vi "1762PointUpProgram.vi"() -> ()   [LabVIEW 2012]
uses:
  <vilib>/Utility/file.llb/Write To Spreadsheet File (DBL).vi
panel:
  out "digital waveform out 3":digitalwaveform(waveform)={"t0"=timestamp(0 s since 1904-01-01), "dt"=1e-07, "Y"={"transitions"=[0, 20000, 21001, 21501, 22501, 42500], "data"=[[1, 1, 0, 0], [0, 0, 0, 0], [0, 0, 0, 1], [0, 0, 0, 0], [1, 1, 0, 0], [1, 1, 0, 0]]}, "error"={"status"=FALSE, "code"=37421928, "source"=""}}
  out "10xwindow":i32
  out "10xdiscr":dbl
  out "DARK?":i32(graph)
  out "Counts":i32
  out "DARK?":bool
  out "PMT Counts":i32(graph)
  in  "PMT sample time":dbl=0.05
  out "Counts after 1762":i32=57
  out "OuterLoop":i32=101
  out "InnerLoop":i32=19
  out "Frequency Step Size":dbl=10000.0
  out "Bright Events":dbl
  in  "Discriminator Level\n (Bright/Dark)":i32=28
  out "digital waveform out 2":digitalwaveform(waveform)={"t0"=timestamp(0 s since 1904-01-01), "dt"=1e-07, "Y"={"transitions"=[0, 20000, 21001, 21501, 22501, 42500], "data"=[[1, 1, 0, 0], [0, 0, 0, 0], [0, 0, 0, 1], [0, 0, 0, 0], [1, 1, 0, 0], [1, 1, 0, 0]]}, "error"={"status"=FALSE, "code"=37421928, "source"=""}}
  in  "1762 pulse length (units of 1 us)":dbl=50.0
  in  "Comment":string="SPAOM, DPAOM = 77 MHz"
  in  "B Field":dbl=2.26
  in  "Power":dbl
  in  "Rerun BG Every\nnth freq point":dbl=20.0
  in  "PMT sample time":dbl=0.05
  out "Counts finding bright ion":dbl=39.0
  in  "BG Cutoff Limit":dbl=38.0
  in  "Runs per data point":dbl=50.0
  in  "Low Freq":dbl(slide)=83600000.0 min=50000000.0 max=120000000.0 step=1000.0 scale=80000000.0..90000000.0 scale format="%#.5f"
  in  "High Freq":dbl(slide)=84100000.0 min=50000000.0 max=120000000.0 step=1000.0 scale=80000000.0..90000000.0 scale format="%#.0f"
  out "Cur Freq":dbl=85984000.0 format="%#_8f"
  out "Path":path=path "c:/data/1762 Scans/2014-05-20_19-16-05_1762scanWithPumping.txt"
  out "Frequency Scan":cluster{dbl, dbl}[](graph)=[{87004000.0, 1.0}, {86994000.0, 1.0}, {86984000.0, 1.0}, {86974000.0, 1.0}, {86964000.0, 1.0}, {86954000.0, 1.0}, {86944000.0, 1.0}, {86934000.0, 1.0}, {86924000.0, 1.0}, {86914000.0, 1.0}, {86904000.0, 1.0}, {86894000.0, 1.0}, {86884000.0, 1.0}, {86874000.0, 1.0}, {86864000.0, 1.0}, {86854000.0, 1.0}, {86844000.0, 1.0}, {86834000.0, 1.0}, {86824000.0, 1.0}, {86814000.0, 1.0}, {86804000.0, 1.0}, {86794000.0, 1.0}, {86784000.0, 1.0}, {86774000.0, 1.0}, {86764000.0, 1.0}, {86754000.0, 1.0}, {86744000.0, 1.0}, {86734000.0, 1.0}, {86724000.0, 1.0}, {86714000.0, 1.0}, {86704000.0, 1.0}, {86694000.0, 1.0}, {86684000.0, 1.0}, {86674000.0, 1.0}, {86664000.0, 1.0}, {86654000.0, 1.0}, {86644000.0, 1.0}, {86634000.0, 1.0}, {86624000.0, 1.0}, {86614000.0, 1.0}, {86604000.0, 1.0}, {86594000.0, 1.0}, {86584000.0, 1.0}, {86574000.0, 1.0}, {86564000.0, 1.0}, {86554000.0, 1.0}, {86544000.0, 1.0}, {86534000.0, 1.0}, {86524000.0, 1.0}, {86514000.0, 1.0}, {86504000.0, 1.0}, {86494000.0, 1.0}, {86484000.0, 1.0}, {86474000.0, 1.0}, {86464000.0, 1.0}, {86454000.0, 1.0}, {86444000.0, 1.0}, {86434000.0, 1.0}, {86424000.0, 1.0}, {86414000.0, 1.0}, {86404000.0, 1.0}, {86394000.0, 1.0}, {86384000.0, 1.0}, {86374000.0, 1.0}, {86364000.0, 1.0}, {86354000.0, 1.0}, {86344000.0, 1.0}, {86334000.0, 1.0}, {86324000.0, 1.0}, {86314000.0, 1.0}, {86304000.0, 1.0}, {86294000.0, 1.0}, {86284000.0, 1.0}, {86274000.0, 1.0}, {86264000.0, 1.0}, {86254000.0, 1.0}, {86244000.0, 1.0}, {86234000.0, 1.0}, {86224000.0, 1.0}, {86214000.0, 1.0}, {86204000.0, 1.0}, {86194000.0, 1.0}, {86184000.0, 1.0}, {86174000.0, 1.0}, {86164000.0, 1.0}, {86154000.0, 1.0}, {86144000.0, 1.0}, {86134000.0, 1.0}, {86124000.0, 1.0}, {86114000.0, 1.0}, {86104000.0, 1.0}, {86094000.0, 1.0}, {86084000.0, 1.0}, {86074000.0, 1.0}, {86064000.0, 1.0}, {86054000.0, 1.0}, {86044000.0, 1.0}, {86034000.0, 1.0}, {86024000.0, 1.0}, {86014000.0, 1.0}, {86004000.0, 1.0}, {85994000.0, 1.0}]
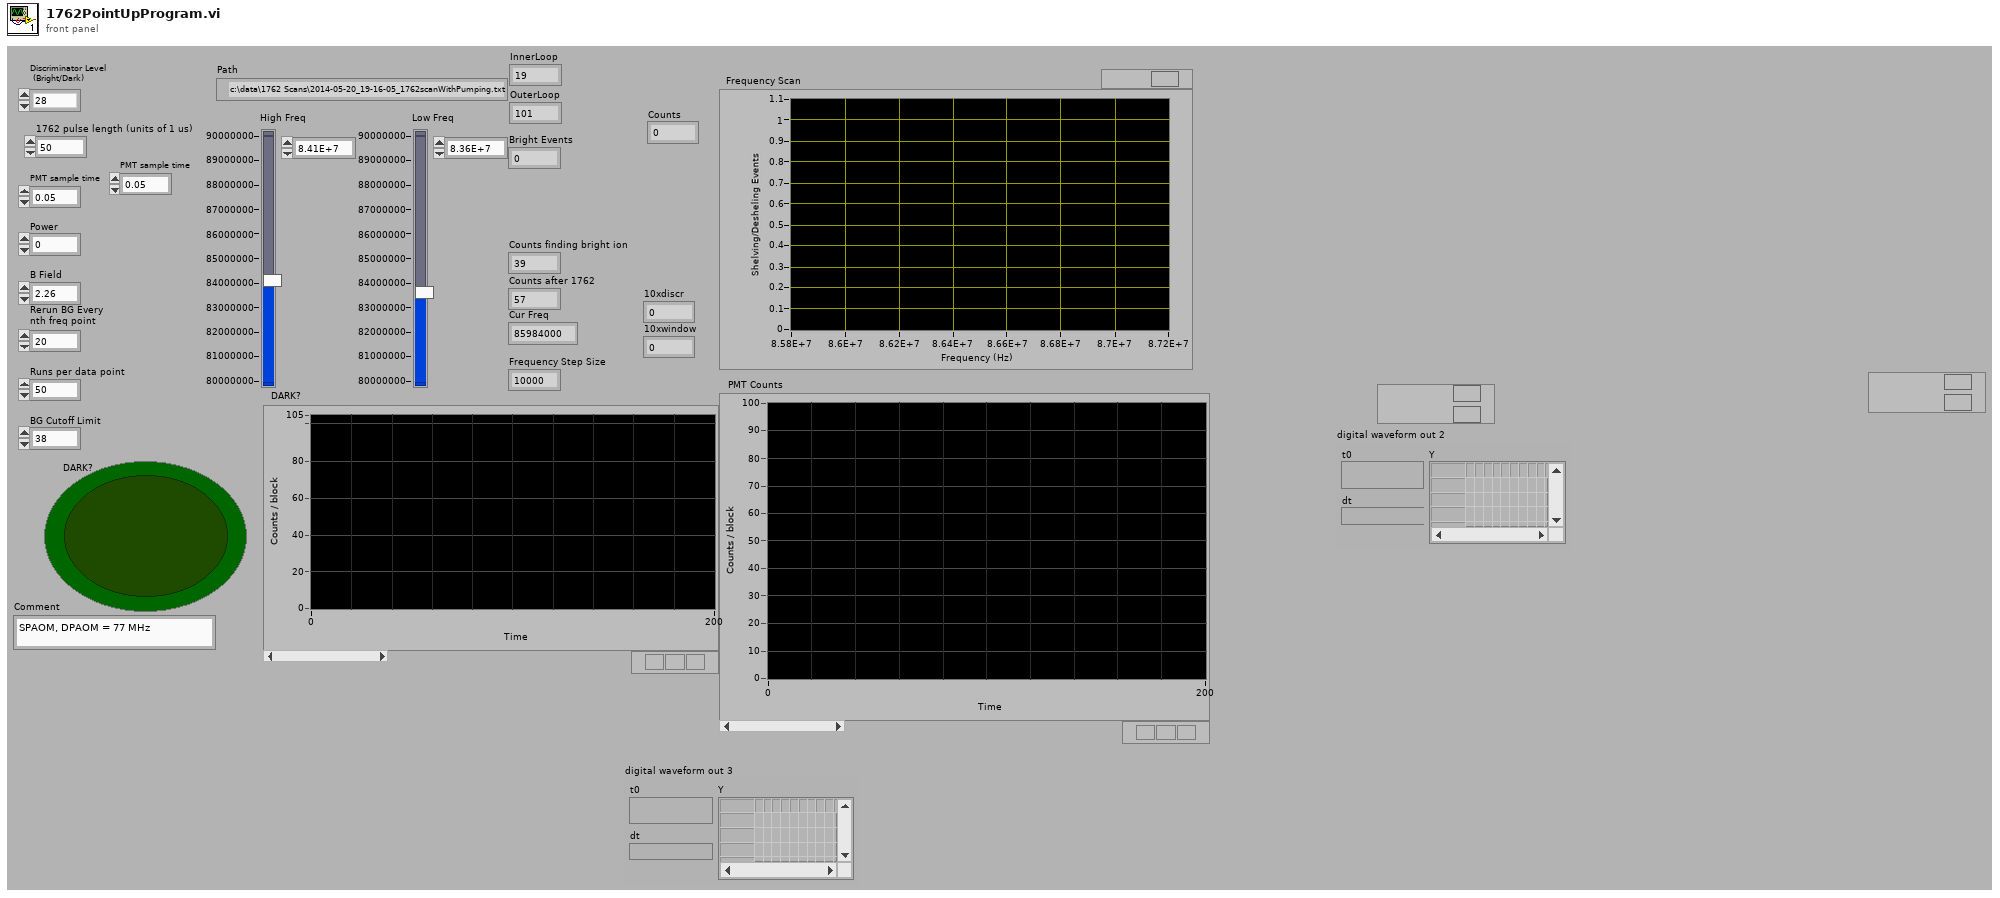
[diagram p1: front panel]
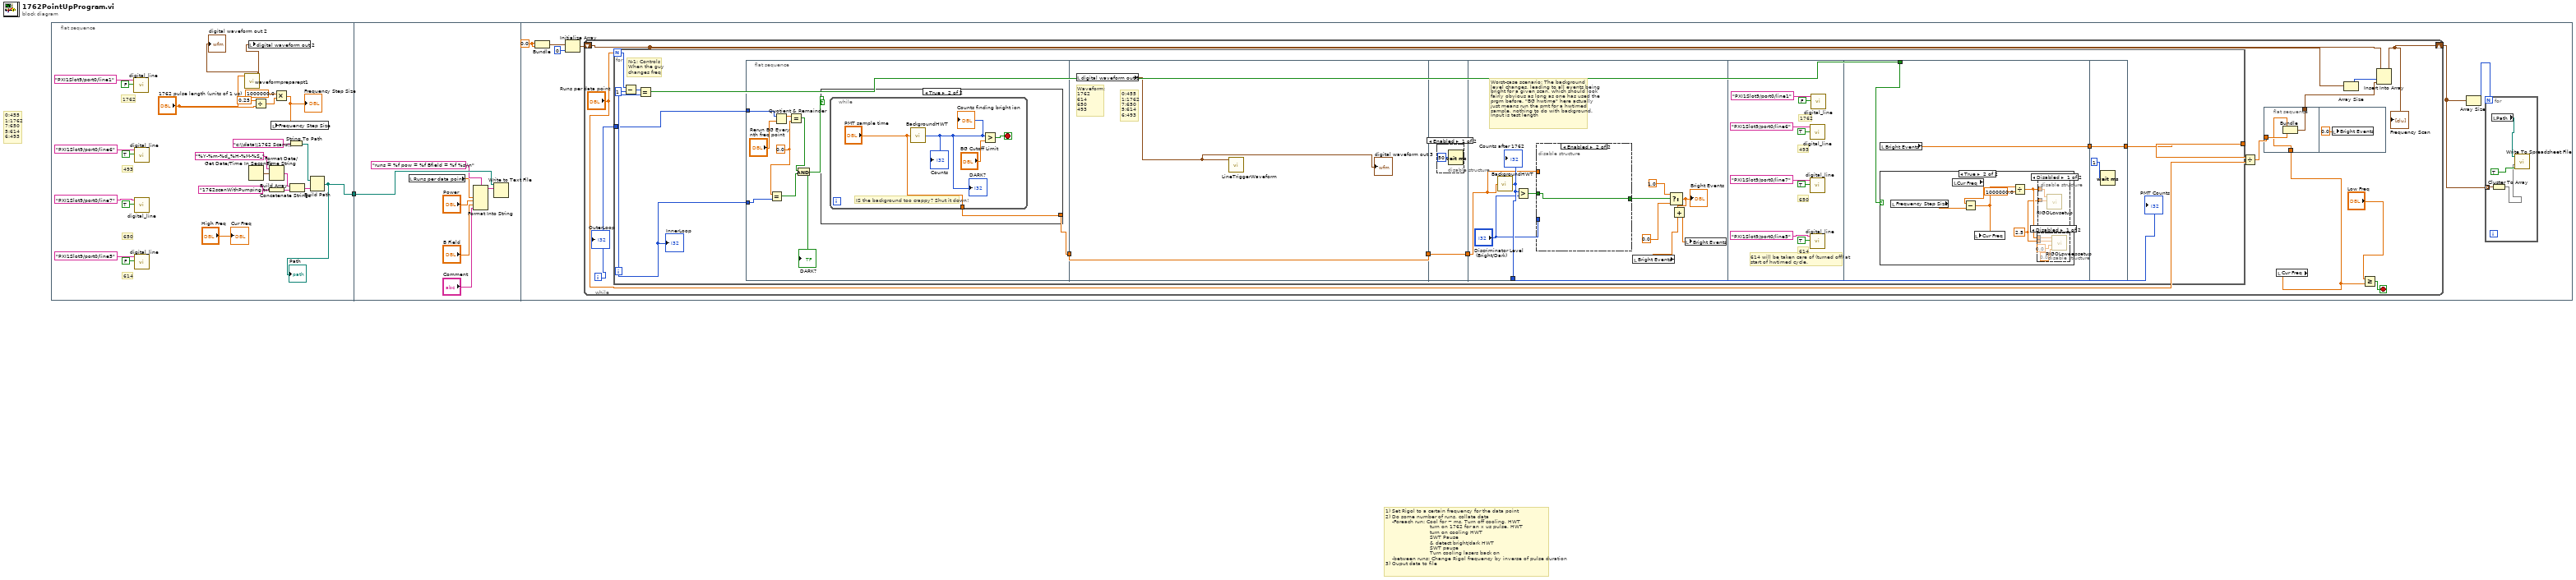
[diagram p0: block diagram]
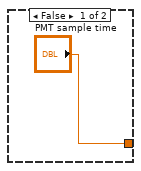
[diagram p2: hidden frame]
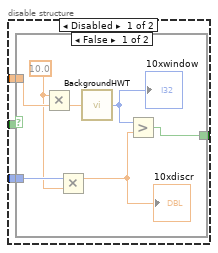
[diagram p4: hidden frame]
diagram:
  # "0:455\n1:1762\n7:650\n5:614\n6:493"
  # "1) Set Rigol to a certain frequency for the data point\n2) Do some number of runs, collate data\n    -Foreach run: Cool for ~ ms, Turn off cooling, HWT\n                           turn on 1762 for an x us pulse, HWT\n                           turn on cooling HWT\n                           SWT Pause\n                           & detect bright/dark HWT\n                           SWT pause\n                           Turn cooling lasers back on \n    -between runs: Change Rigol frequency by inverse of pulse duration\n3) Ouput data to file"
  n1 = flat-sequence {
    tunnel: [w17] -> w1
    tunnel: w1 -> [w32]
    frame #0 {
      # "614"
      # "650"
      # "493"
      # "1762"
      n2 = call "digital_line.vi"("Boolean"=FALSE, "lines"=tag "PXI1Slot9/port0/line1") -> ()  [unwired: 5 in, 1 out]
      n3 = call "digital_line.vi"("Boolean"=TRUE, "lines"=tag "PXI1Slot9/port0/line6") -> ()  [unwired: 5 in, 1 out]
      n4 = call "digital_line.vi"("Boolean"=TRUE, "lines"=tag "PXI1Slot9/port0/line7") -> ()  [unwired: 5 in, 1 out]
      n5 = call "digital_line.vi"("Boolean"=FALSE, "lines"=tag "PXI1Slot9/port0/line5") -> ()  [unwired: 5 in, 1 out]
      n6 = call "waveformpreparept1.vi"("1762 pulse length (units of 1 us)"="1762 pulse length (units of 1 us)") -> ("digital waveform out 2"=w2:digitalwaveform)  [unwired: 8 in]
      "digital waveform out 2" <- w2
      n7 = local write "digital waveform out 2"(w2) -> ()
      n8 = Get Date/Time In Seconds() -> (seconds since 1Jan1904=w19:timestamp)
      n9 = Divide(x=0.25, y="1762 pulse length (units of 1 us)") -> (x/y=w5:dbl)
      n10 = Format Date/Time String(time format string (%c)="%Y-%m-%d_%H-%M-%S_", seconds (now)=w19) -> (date/time string=w21:string)  [unwired: 1 in]
      n11 = Build Array("1762scanWithPumping.txt") -> (w24:string[])
      n12 = Multiply(x=1000000.0, y=w5) -> (x*y=w6:dbl)
      "Frequency Step Size" <- w6
      n13 = local write "Frequency Step Size"(w6) -> ()
      n14 = String To Path(string="c:\\data\\1762 Scans\\") -> (path=w25:path)
      n15 = Concatenate Strings(w21, w24) -> (w23:string)
      n16 = Build Path(base path=w25, name or relative path=w23) -> (appended path=w17:path)
      "Path" <- w17
      "Cur Freq" <- "High Freq"
    }
    frame #1 {
      n17 = local read "Runs per data point"() -> (w29:dbl)
      n18 = Format Into String(format string="runs = %f pow = %f Bfield = %f %s\\n", w29, "Power", "B Field", "Comment") -> (resulting string=w30:string)  [unwired: 2 in, 1 out]
      n19 = Write to Text File(file (use dialog)=w32, text=w30) -> ()  [unwired: 2 in, 3 out]
    }
    frame #2 {
      w37 = 0.0
      n20 = Bundle(w37, w37) -> (w38:cluster{dbl, dbl})  [unwired: 1 in]
      n21 = Initialize Array(w38, 0) -> (w35:cluster{dbl, dbl}[])
      n22 = while {
        shift-right: [w49] -> w33
        shift-left: w35 -> [w50]
        i -> [w48]
        stop <- w52 stop-if-true
        n23 = for {
          N: "Runs per data point" -> [w66]
          tunnel: [w65] -> w45
          tunnel: w48 -> [w62]
          i -> [w63]
          # "N-1: Controls\nWhen the guy\nchanges freq"
          n24 = Subtract(x=w66, y=1) -> (x-y=w69:i32)
          n25 = Equal?(x=w69, y=w63) -> (x = y?=w67:bool)
          n26 = flat-sequence {
            tunnel: w63 -> [w76]
            tunnel: w62 -> [w71]
            tunnel: [w70] -> w61
            tunnel: [w86] -> w58
            tunnel: w61 -> [w86]
            tunnel: [w87] -> w59
            tunnel: w58 -> [w87]
            tunnel: w59 -> [w91]
            tunnel: [w93] -> w60
            tunnel: w67 -> [w120]
            tunnel: [w121] -> w64
            tunnel: [w135] -> w65
            tunnel: w64 -> [w135]
            frame #0 {
              w75 = 0.0 ("x")
              n27 = Equal?(x=w75, y=w76) -> (x = y?=w73:bool)
              n28 = Quotient & Remainder(x=w71, y="Rerun BG Every\nnth freq point") -> (x-y*floor(x/y)=w77:dbl)  [unwired: 1 out]
              n29 = Equal?(x=w77, y=w75) -> (x = y?=w74:bool)
              n30 = And(x=w74, y=w73) -> (x .and. y?=w72:bool)
              "DARK?" <- w72
              n31 = case shown="True" w72 {
                tunnel: ["PMT sample time" w80] -> w70
                frame False {
                }
                frame True {
                  n32 = while {
                    tunnel: ["PMT sample time"] -> w80
                    stop <- w83 stop-if-true
                    # "IS the background too crappy? Shut it down!"
                    n33 = call "BackgroundHWT.vi"("Sample Time(seconds)"="PMT sample time") -> ("Counts"=w81:i32)
                    "Counts finding bright ion" <- w81
                    "Counts" <- w81
                    "DARK?" <- w81
                    n34 = Greater?(x=w81, y="BG Cutoff Limit") -> (0:w83:bool)
                  }
                }
              }
            }
            frame #1 {
              # "0:455\n1:1762\n7:650\n5:614\n6:493"
              # "Waveform:\n1762\n614\n650\n493"
              n35 = local read "digital waveform out 2"() -> (w85:digitalwaveform)
              "digital waveform out 3" <- w85
              n36 = call "LineTriggerWaveform.vi"("digital waveform in"=w85) -> ()  [unwired: 11 in]
            }
            frame #2 {
              n37 = disable-structure shown="Enabled" {
                frame Enabled {
                  n38 = Wait (ms)(milliseconds to wait=u32 50) -> ()  [unwired: 1 out]
                }
                frame Disabled {
                }
              }
            }
            frame #3 {
              # "Worst-case scenario: The background\nlevel changes, leading to all events being\nbright for a given scan, which should look\nfairly obvious as long as one has used the\nprgm before. \"BG hwtime\" here actually\njust means run the pmt for a hwtimed\nsample, nothing to do with background.\nInput is test length"
              n39 = call "BackgroundHWT.vi"("Sample Time(seconds)"=w91) -> ("Counts"=w93:i32)
              "Counts after 1762" <- w93
              n40 = Greater?(x=w93, y="Discriminator Level\n (Bright/Dark)") -> (0:w92:bool)
              n41 = disable-structure shown="Enabled" {
                disable-tunnel: w92 -> [w102 w111]
                disable-tunnel: [w101 w111] -> w89
                disable-tunnel: w91 -> [w100 _]
                disable-tunnel: "Discriminator Level\n (Bright/Dark)" -> [w99 _]
                frame Disabled {
                  n42 = case shown="False" w102 {
                    selector: w102 -> [_ w110]
                    tunnel: [w105 w110] -> w101
                    tunnel: w100 -> [w109 _]
                    tunnel: w99 -> [w106 _]
                    frame False {
                      w103 = 10.0 ("x")
                      n43 = Multiply(x=w103, y=w109) -> (x*y=w108:dbl)
                      n44 = Multiply(x=w106, y=w103) -> (x*y=w104:dbl)
                      "10xdiscr" <- w104
                      n45 = call "BackgroundHWT.vi"("Sample Time(seconds)"=w108) -> ("Counts"=w107:i32)
                      "10xwindow" <- w107
                      n46 = Greater?(x=w107, y=w104) -> (0:w105:bool)
                    }
                    frame True {
                    }
                  }
                }
                frame Enabled {
                }
              }
              n47 = local read "Bright Events"() -> (w94:dbl)
              n48 = Select(t=1.0, s=w89, f=0.0) -> (s? t:f=w96:dbl)
              "Bright Events" <- w96
              n49 = Add(x=w96, y=w94) -> (x+y=w95:dbl)
              n50 = local write "Bright Events"(w95) -> ()
            }
            frame #4 {
              # "614 will be taken care of (turned off) at\nstart of hwtimed cycle."
              # "614"
              # "650"
              # "493"
              # "1762"
              n51 = call "digital_line.vi"("Boolean"=TRUE, "lines"=tag "PXI1Slot9/port0/line6") -> ()  [unwired: 5 in, 1 out]
              n52 = call "digital_line.vi"("Boolean"=TRUE, "lines"=tag "PXI1Slot9/port0/line7") -> ()  [unwired: 5 in, 1 out]
              n53 = call "digital_line.vi"("Boolean"=TRUE, "lines"=tag "PXI1Slot9/port0/line5") -> ()  [unwired: 5 in, 1 out]
              n54 = call "digital_line.vi"("Boolean"=FALSE, "lines"=tag "PXI1Slot9/port0/line1") -> ()  [unwired: 5 in, 1 out]
            }
            frame #5 {
              n55 = case shown="True" w120 {
                frame False {
                }
                frame True {
                  w122 = 2.5 ("Amplitude (Vpp)")
                  n56 = local read "Frequency Step Size"() -> (w126:dbl)
                  n57 = local read "Cur Freq"() -> (w127:dbl)
                  n58 = Subtract(x=w127, y=w126) -> (x-y=w125:dbl)
                  n59 = local write "Cur Freq"(w125) -> ()
                  n60 = Divide(x=w125, y=1000000.0) -> (x/y=w123:dbl)
                  n61 = disable-structure shown="Disabled" {
                    disable-tunnel: w123 -> [w129 _]
                    disable-tunnel: w122 -> [w128 _]
                    frame Disabled {
                      n62 = call "RIGOLsweepsetup.vi"("AP Sweep Width (MHz)"=0.0, "Time (ms)"=0.0, "Amplitude (Vpp)"=w128, "Frequency (MHz)"=w129) -> ()  [unwired: 8 in]
                    }
                    frame Enabled {
                    }
                  }
                  n63 = disable-structure shown="Disabled" {
                    disable-tunnel: w122 -> [w133 _]
                    disable-tunnel: w123 -> [w132 _]
                    frame Disabled {
                      n64 = call "RIGOLcwsetup.vi"("Amplitude (Vpp)"=w133, "Frequency (MHz)"=w132) -> ()  [unwired: 10 in]
                    }
                    frame Enabled {
                    }
                  }
                }
              }
              n65 = local read "Bright Events"() -> (w121:dbl)
            }
            frame #6 {
              n66 = Wait (ms)(milliseconds to wait=u32 1) -> ()  [unwired: 1 out]
            }
          }
          "InnerLoop" <- w63
          "PMT Counts" <- w60
        }
        n67 = Divide(x=w45, y="Runs per data point") -> (x/y=w44:dbl)
        n68 = flat-sequence {
          tunnel: w44 -> [w56]
          tunnel: [w55] -> w47
          tunnel: w46 -> [w54]
          frame #0 {
            n69 = Bundle("Cur Freq"=w54, w56) -> (w55:cluster{"Cur Freq":dbl, dbl})  [unwired: 1 in]
          }
          frame #1 {
            n70 = local write "Bright Events"(0.0 ("Bright Events")) -> ()
          }
        }
        n71 = local read "Cur Freq"() -> (w46:dbl)
        n72 = Array Size(array=w50) -> (size(s)=w51:i32)
        n73 = Greater Or Equal?(x="Low Freq", y=w46) -> (x >= y?=w52:bool)
        n74 = Insert Into Array(array=w50, index=w51, new element=w47) -> (w49:cluster{dbl, dbl}[])
        "Frequency Scan" <- w49
        "OuterLoop" <- w48
      }
      n75 = Array Size(array=w33) -> (size(s)=w34:i32)
      n76 = for {
        N: w34 -> [_]
        tunnel: w33 -> [w42] mode=indexing
        n77 = local read "Path"() -> (w39:path)
        n78 = Cluster To Array(cluster=w42) -> (array=w40:dbl[])
        n79 = call-poly <vilib>:"Write To Spreadsheet File.vi"("append to file? (new file:F)"=TRUE, "1D data"=w40, "file path (dialog if empty)"=w39) -> ()  [unwired: 5 in, 1 out]
      }
    }
  }
